vi "Cal16Bit.vi"   [LabVIEW 2014]
uses:
  ESLSCDLL.dll
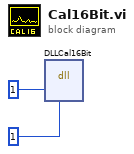
[diagram p0: block diagram]
diagram:
  n1 = dll-call lib="C:/Users/Gerhard/Documents/New64/lv/1cam/board.vis/ESLSCDLL.dll" fn="DLLCal16Bit"("drv"=u32 1, "zadr"=u32 1) -> ()  [unwired: 6 in, 2 out]
